vi "ADD RECORD消息解析.vi"(9 "body":string, 11 "消息框":refnum<vi>) -> ()   [LabVIEW 2015]
uses:
  Global.vi
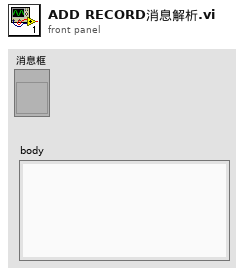
[diagram p1: front panel]
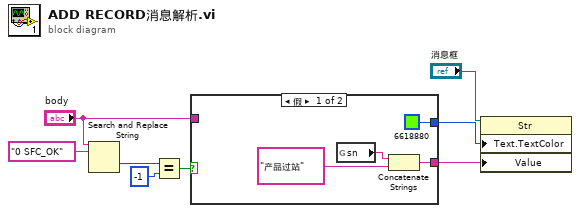
[diagram p0: block diagram]
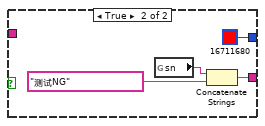
[diagram p2: hidden frame]
diagram:
  n1 = Search and Replace String(input string="body", search string="0 SFC_OK") -> (offset past replacement=w7:i32)  [unwired: 6 in, 3 out]
  n2 = Equal?(x=w7, y=-1) -> (x = y?=w4:bool)
  n3 = case shown="假" w4 {
    tunnel: [w12 w13] -> w3
    tunnel: [u32 6618880 u32 16711680] -> w2
    tunnel: "body" -> [_ _]
    frame False {
      n4 = global read "Global.vi" "sn"() -> (w9:string)
      n5 = Concatenate Strings(w9, "产品过站") -> (w12:string)
    }
    frame True {
      n6 = global read "Global.vi" "sn"() -> (w15:string)
      n7 = Concatenate Strings(w15, "测试NG") -> (w13:string)
    }
  }
  n8 = property class="Str"(reference="消息框", "Text.TextColor"=w2, "Value"=w3) -> ()  [unwired: 1 in, 2 out]
